vi "FT10_M4X Read Data.vi"(0 "Card Handle in":u32, 5 "Offset (Samples per Channel)":u32, 7 "Length (Samples per Channel)":u32, 9 "Channel Count":u32) -> (4 "Card Handle out":u32, 6 "Ch 0":sgl[](array[numeric]) format="%.2f", 8 "Ch 1":sgl[](array[numeric]) format="%.2f", 10 "Ch 2":sgl[](array[numeric]) format="%.2f", 15 "Ch 3":sgl[](array[numeric]) format="%.2f")   [LabVIEW 2024]
doc: "Copy of \"M4X_Read_Data.vi\" from HWT_Lillis_7854.lvproj"
uses:
  LV2015/Transfer dlls/spcm_datasort_win32.dll
panel:
  # "This Vi reads out sorted channel data for card that have between 1 and 16 analog channels. \nThe data is converted to float values of voltage including the currently set input range and the \ncurrent programmed offset for each channel. \n\nThis is an universal sorting VI. Please specify the number of channels to be sorted and connect\nall output channels that you use"
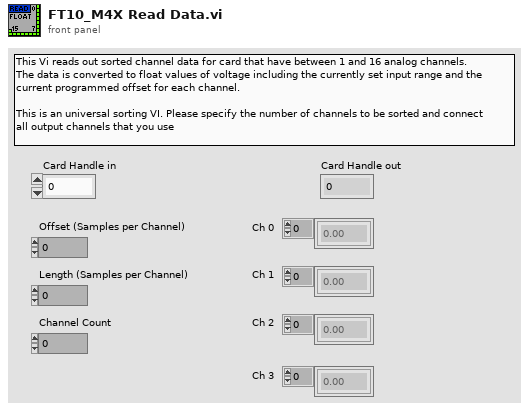
[diagram p1: front panel]
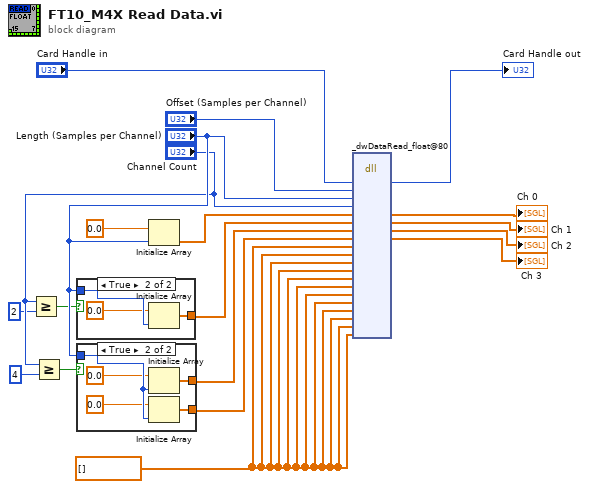
[diagram p0: block diagram]
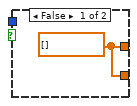
[diagram p2: hidden frame]
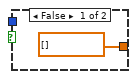
[diagram p3: hidden frame]
diagram:
  w16 = sgl[] []
  n1 = Greater Or Equal?(x="Channel Count", y=u32 2) -> (x >= y?=w2:bool)
  n2 = Greater Or Equal?(x="Channel Count", y=u32 4) -> (x >= y?=w9:bool)
  n3 = case shown="True" w2 {
    tunnel: [sgl[] [] w23] -> w5
    tunnel: "Length (Samples per Channel)" -> [_ w22]
    frame False {
    }
    frame True {
      n4 = Initialize Array(sgl 0.0, w22) -> (w23:sgl[])
    }
  }
  n5 = case shown="True" w9 {
    tunnel: [w24 w29] -> w6
    tunnel: "Length (Samples per Channel)" -> [_ w27]
    tunnel: [w24 w28] -> w7
    frame False {
      w24 = sgl[] []
    }
    frame True {
      n6 = Initialize Array(sgl 0.0, w27) -> (w29:sgl[])
      n7 = Initialize Array(sgl 0.0, w27) -> (w28:sgl[])
    }
  }
  n8 = Initialize Array(sgl 0.0, "Length (Samples per Channel)") -> (w4:sgl[])
  n9 = dll-call lib="C:/Users/yearon2/OneDrive - Medtronic PLC/LV2015/Transfer dlls/spcm_datasort_win32.dll" fn="_dwDataRead_float@80"("hDrv"="Card Handle in", "dwOffset"="Offset (Samples per Channel)", "dwLen"="Length (Samples per Channel)", "dwChCount"="Channel Count", "pfData_Ch0"=w4, "pfData_Ch1"=w5, "pfData_Ch2"=w6, "pfData_Ch3"=w7, "pfData_Ch4"=w16, "pfData_Ch5"=w16, "pfData_Ch6"=w16, "pfData_Ch7"=w16, "pfData_Ch8"=w16, "pfData_Ch9"=w16, "pfData_Ch10"=w16, "pfData_Ch11"=w16, "pfData_Ch12"=w16, "pfData_Ch13"=w16, "pfData_Ch14"=w16, "pfData_Ch15"=w16) -> ("hDrv"=→"Card Handle out":u32, "pfData_Ch0"=→"Ch 0":sgl[], "pfData_Ch1"=→"Ch 1":sgl[], "pfData_Ch2"=→"Ch 2":sgl[], "pfData_Ch3"=→"Ch 3":sgl[])  [unwired: 19 in, 2 out]
